vi "GUI_HTT_Switcher_tester.vi"() -> ()   [LabVIEW 2013]
uses:
  Shared/GUI_Template/GUI_master/tcp_new_data_event.ctl
  Shared/GUI_Template/GUI_master/tcp new data cluster.ctl
panel:
  in  "DigitalOutput.Channel 2::1":enum16{"on", "off"}(ring) caption="Phosphor"
  in  "Phosphor":bool
  in  "DigitalOutput.Channel 1::1":enum16{"on", "off"}(ring)
  in  "DigitalOutput.Channel 0::1":enum16{"on", "off"}(ring) caption="Flipper"
  in  "Flipper":bool
  out "error IO 2":errorcluster
  out "fire::10":string
  out "tcp data event":T1
  in  "UDP error message":string
  in  "GUIdevice 2":string
  in  "GUIdevice 1":string="HTT-Switch-DAQPad"
  in  "stop":bool
  # "Energy"
  # "HTT Switcher"
  # "In"
  # "Out"
  # "In"
  # "Out"
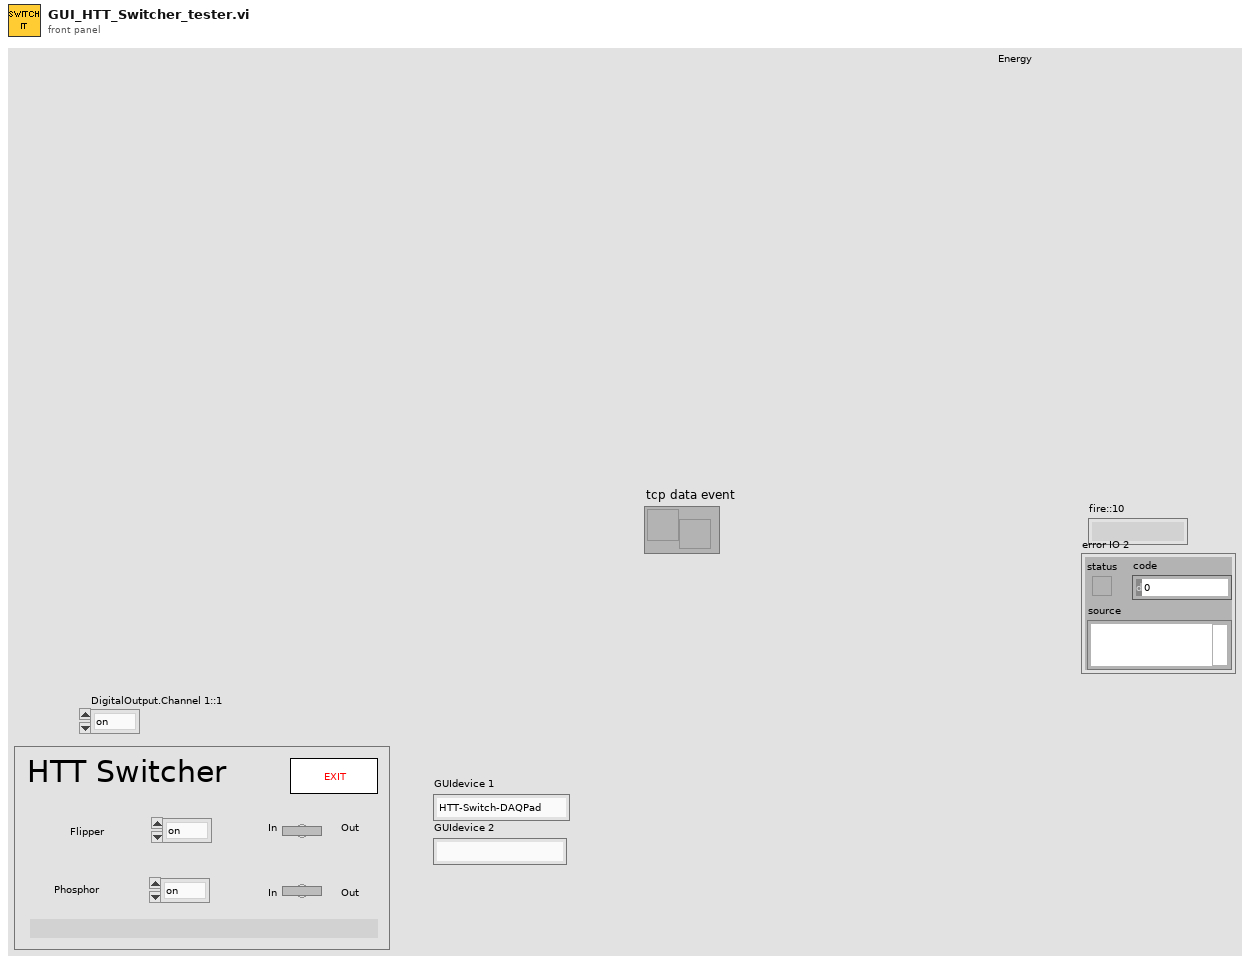
[diagram p1: front panel]
types:
  T1 = typedef "tcp_new_data_event.ctl" = refnum<user-event>
  T2 = typedef "tcp new data cluster.ctl" = cluster{"EventEnum":enum16{"new data", "connection status update"}, "Device name":string}
  T3 = enum32{"invalid app kind", "Development System", "Run Time System", "Student Edition", "Embedded LabVIEW", "Evaluation", "Custom"}
  T4 = enum32{"Invalid", "Standard", "Closed", "Hidden", "Minimized", "Maximized"}
  T5 = cluster{"Core":cluster{"Current VI Reference":refnum<vi>, "Close Panel on Exit?":bool}, "Heater timing offset":dbl, "Discharge timing offset":dbl, "irrelevant":bool, "Tik1":u32, "Tik2":u32, "notused":bool, "outoforder":bool, "notwhatyouthinkitis":enum16{"on", "off"}}
  T6 = cluster{"Current VI Reference":refnum<vi>, "Close Panel on Exit?":bool}
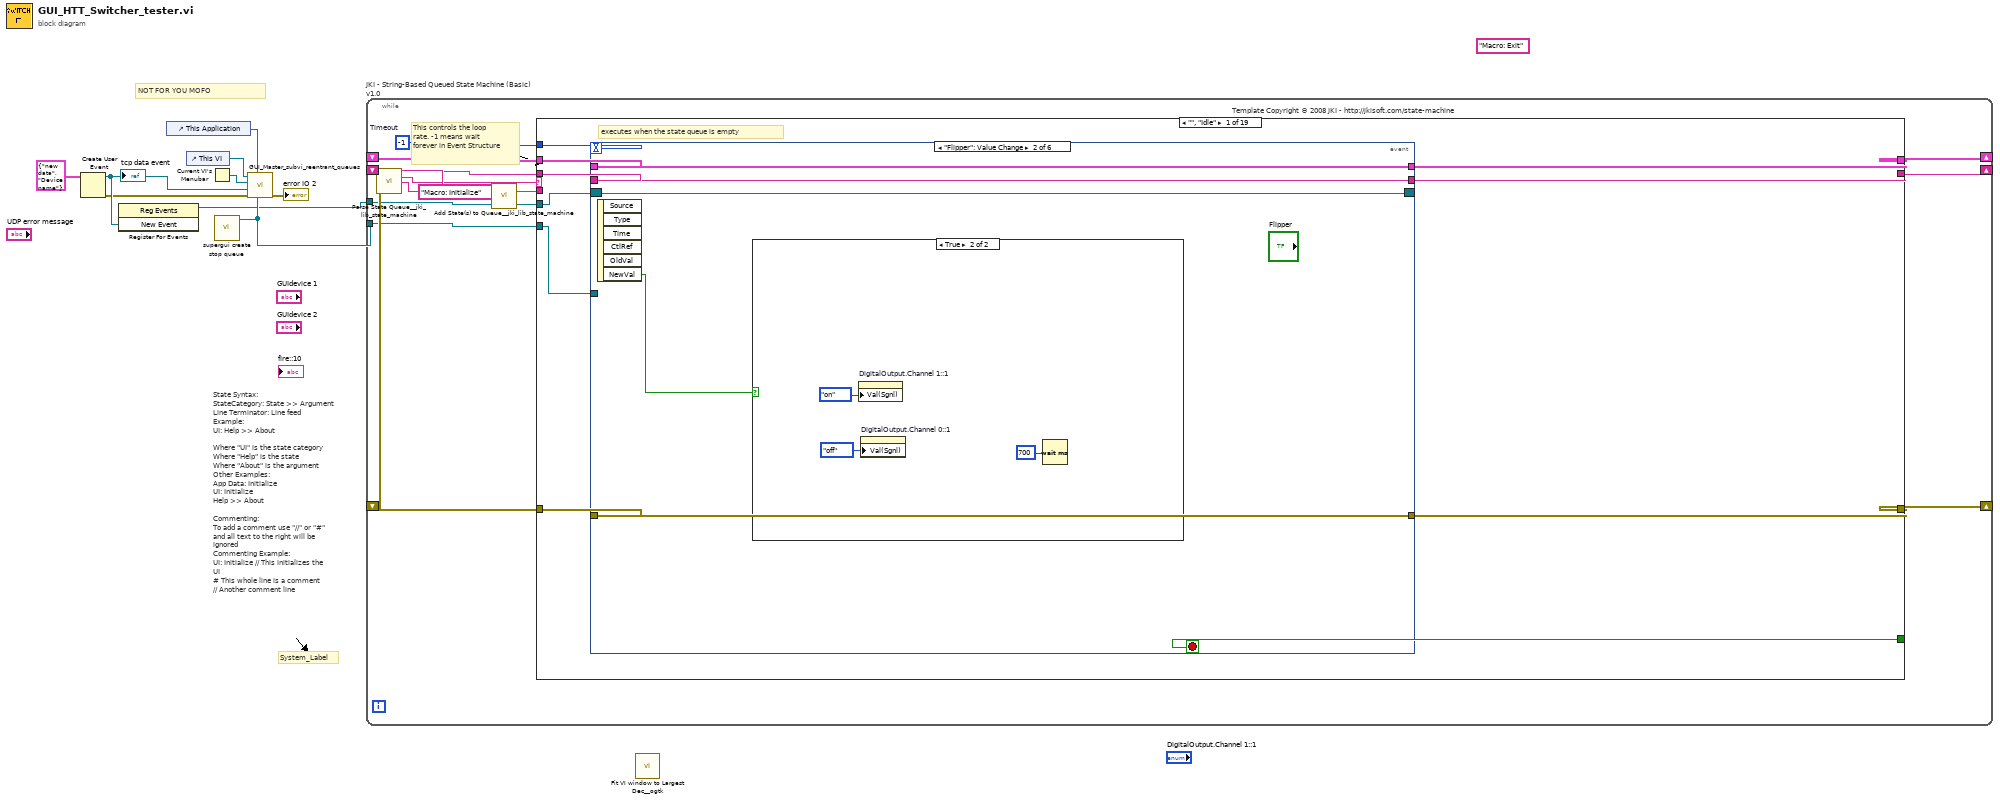
[diagram p0: block diagram]
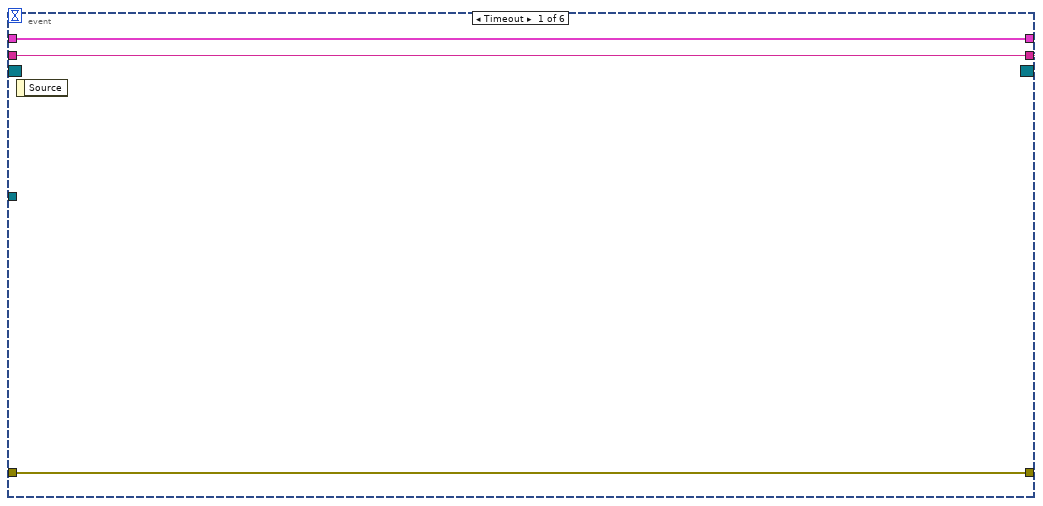
[diagram p2: hidden frame]
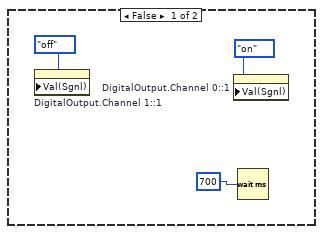
[diagram p3: hidden frame]
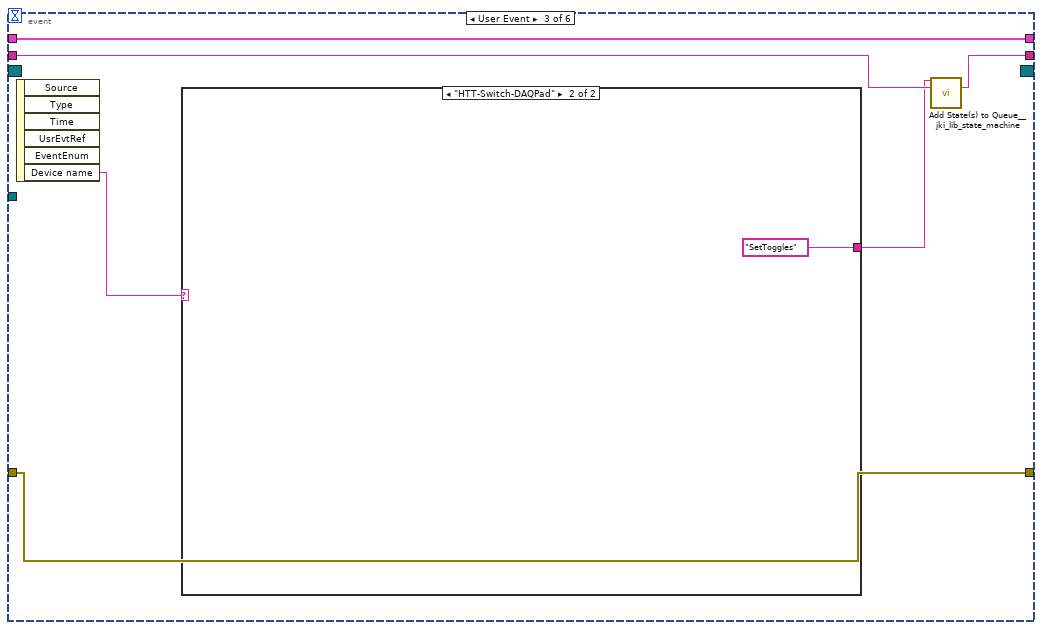
[diagram p4: hidden frame]
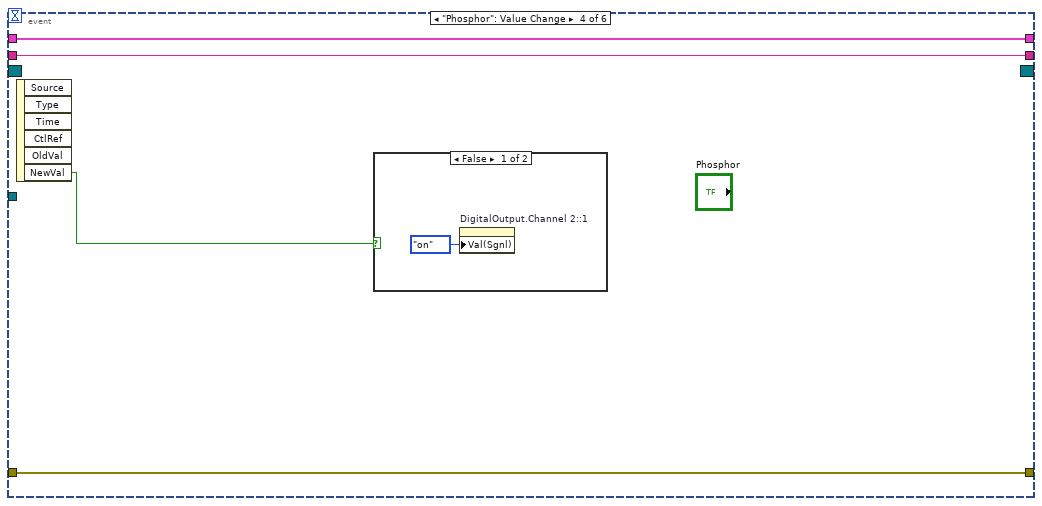
[diagram p6: hidden frame]
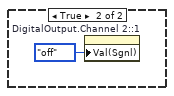
[diagram p7: hidden frame]
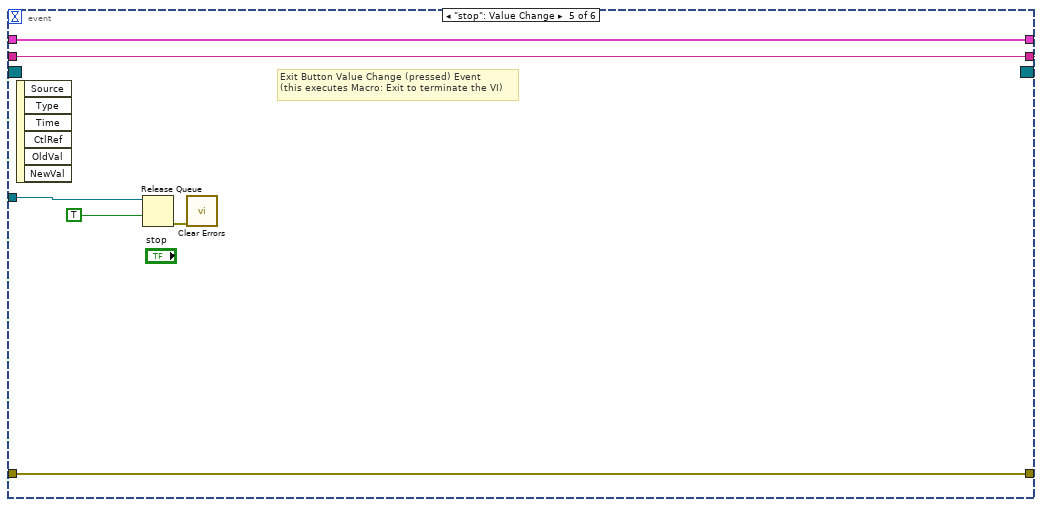
[diagram p8: hidden frame]
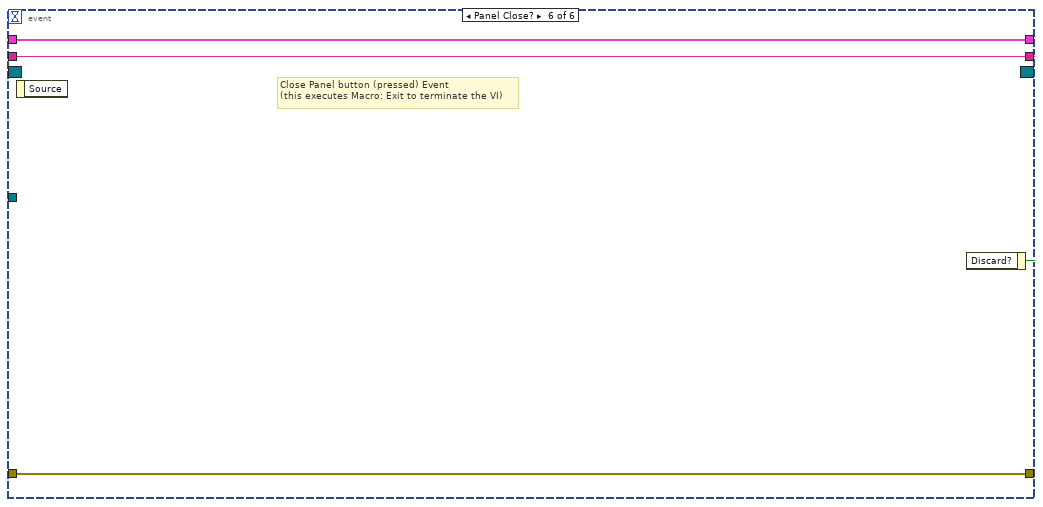
[diagram p9: hidden frame]
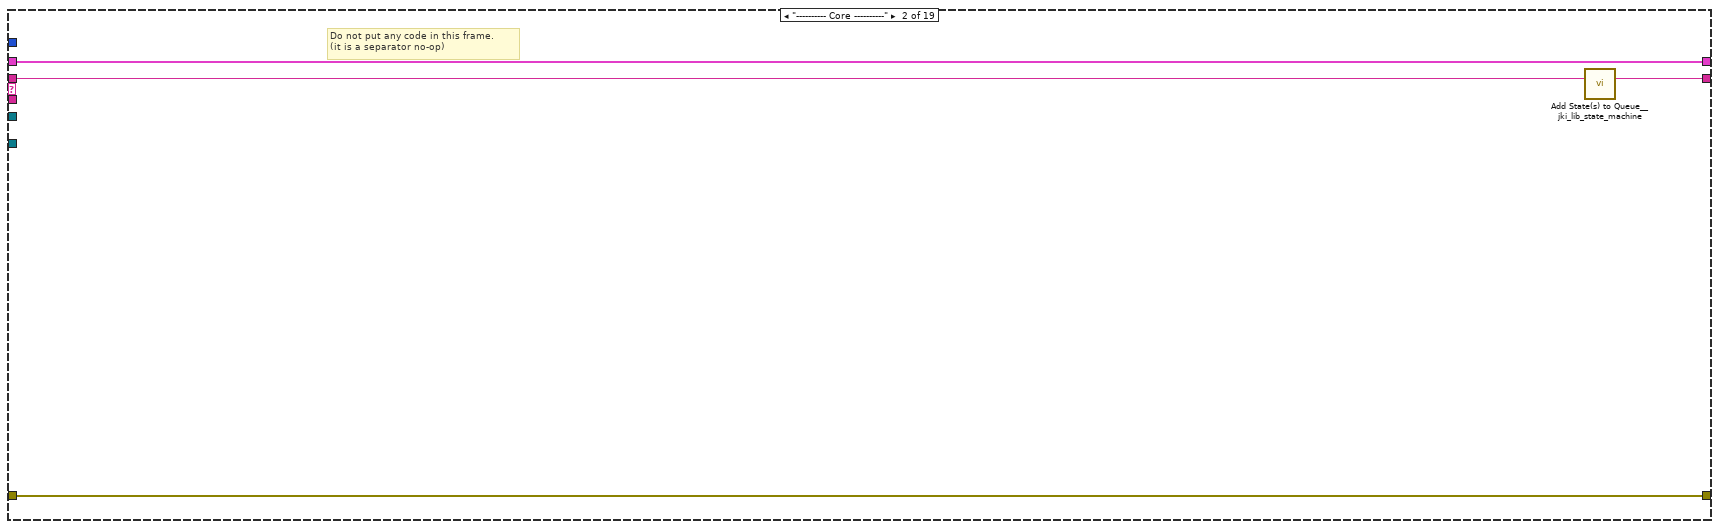
[diagram p10: hidden frame]
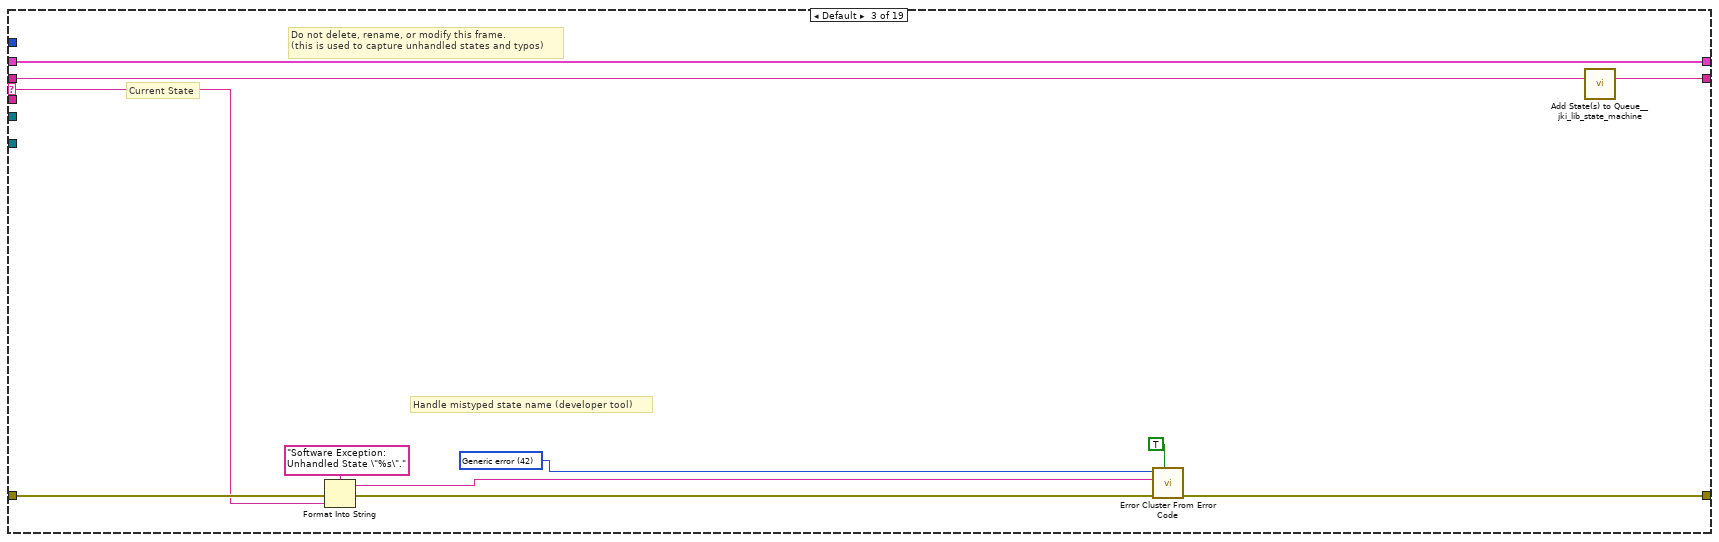
[diagram p11: hidden frame]
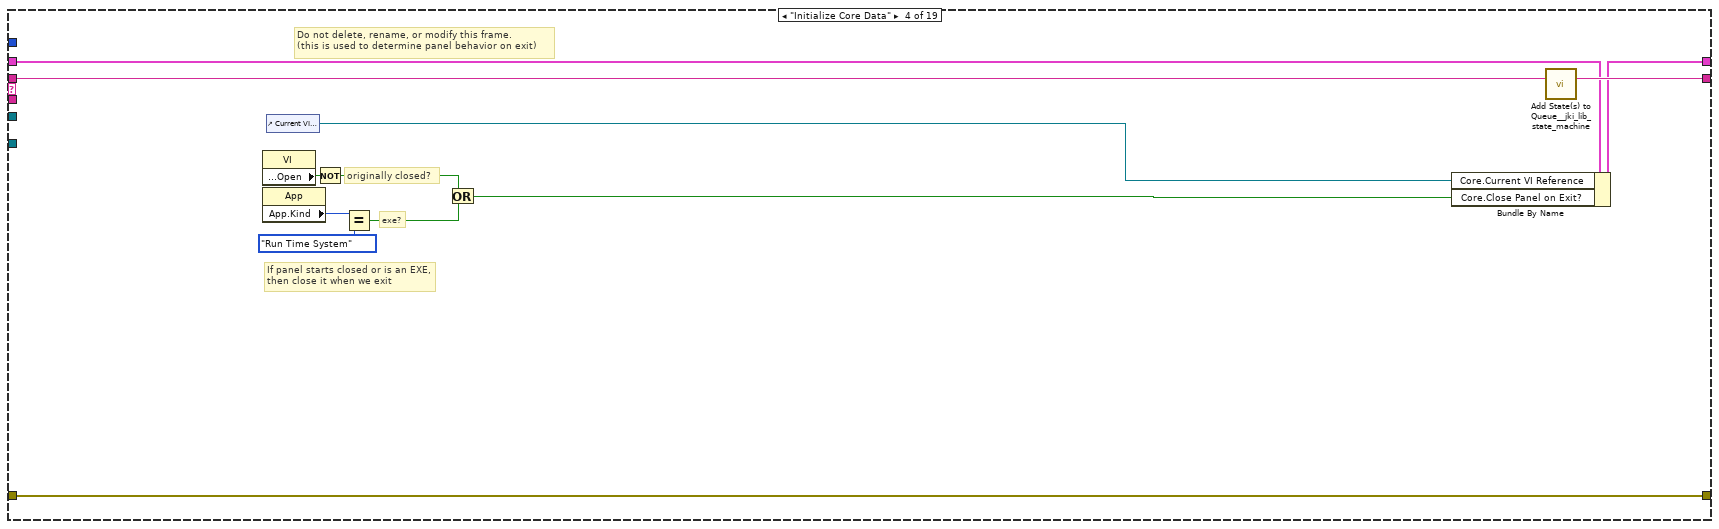
[diagram p12: hidden frame]
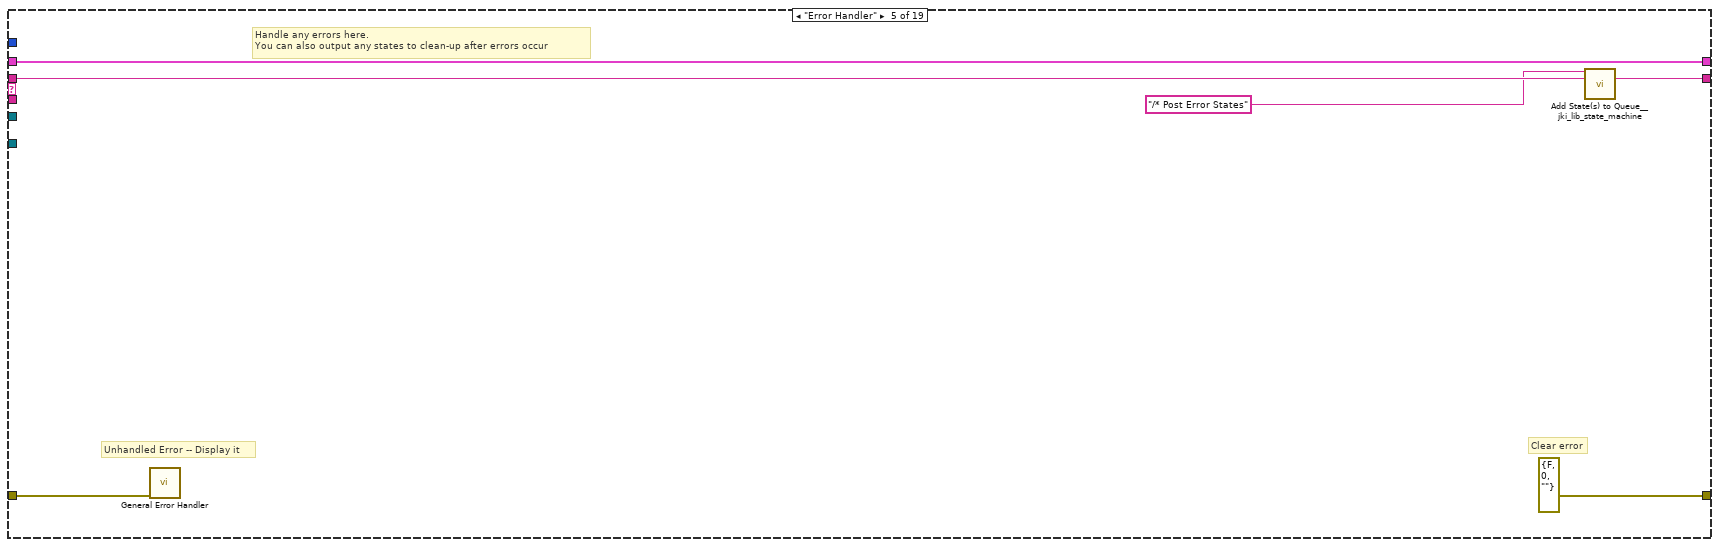
[diagram p13: hidden frame]
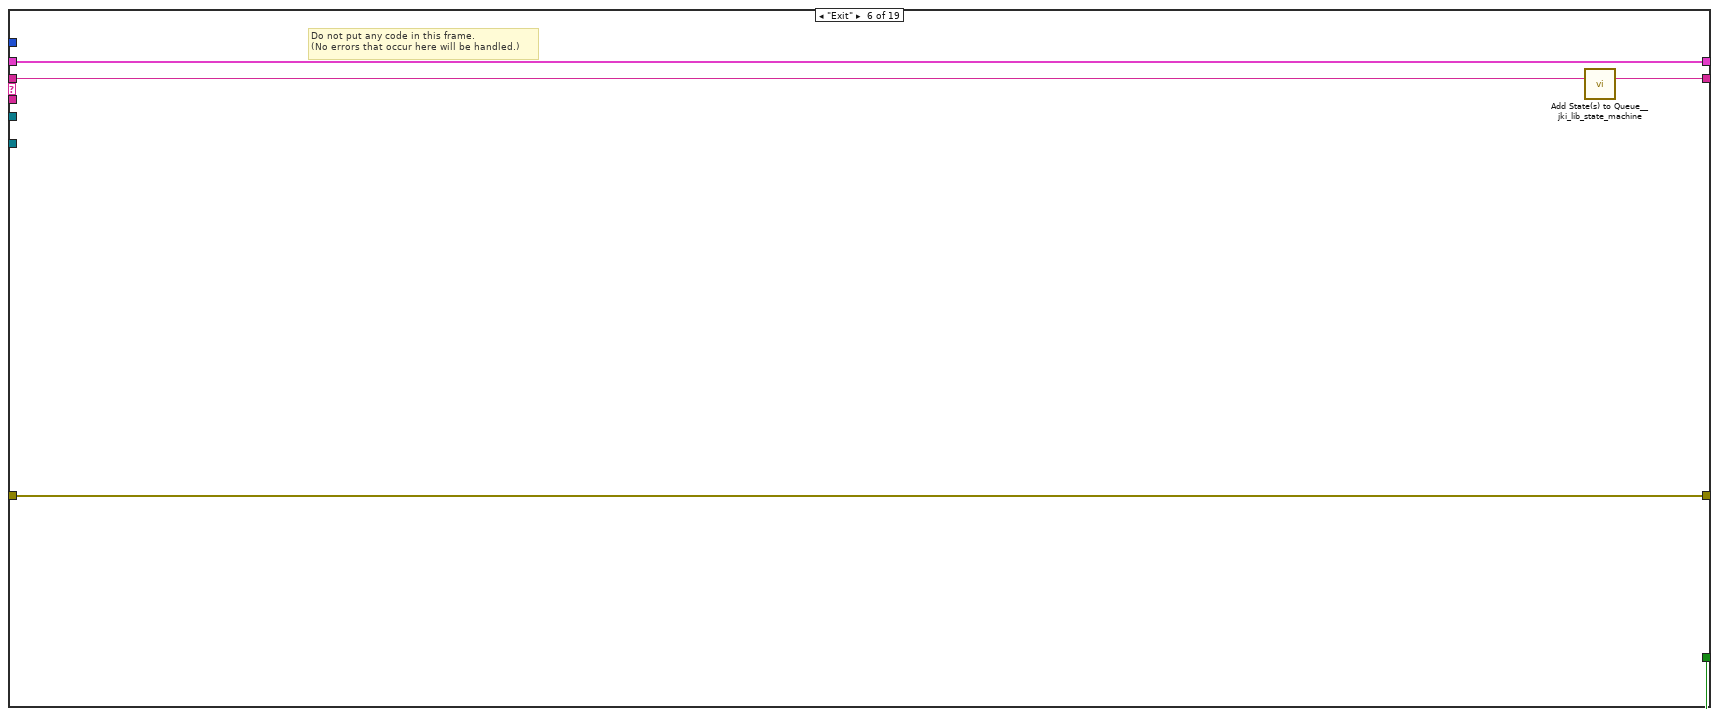
[diagram p14: hidden frame]
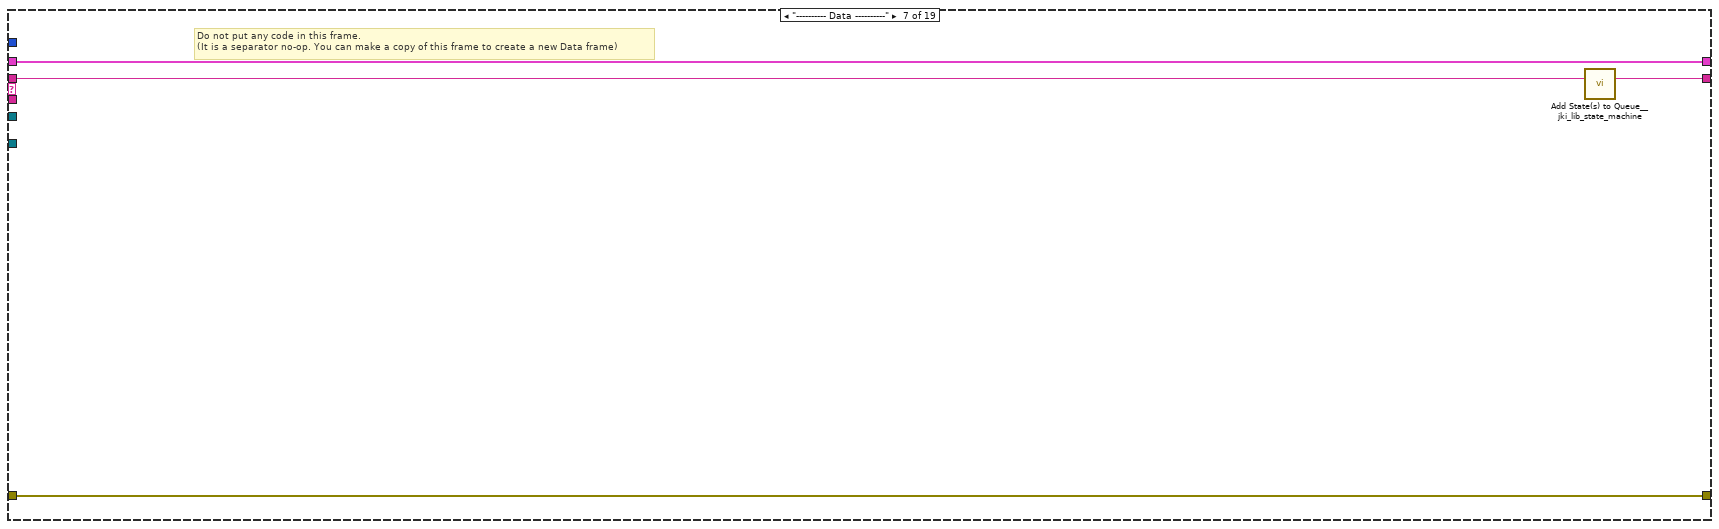
[diagram p15: hidden frame]
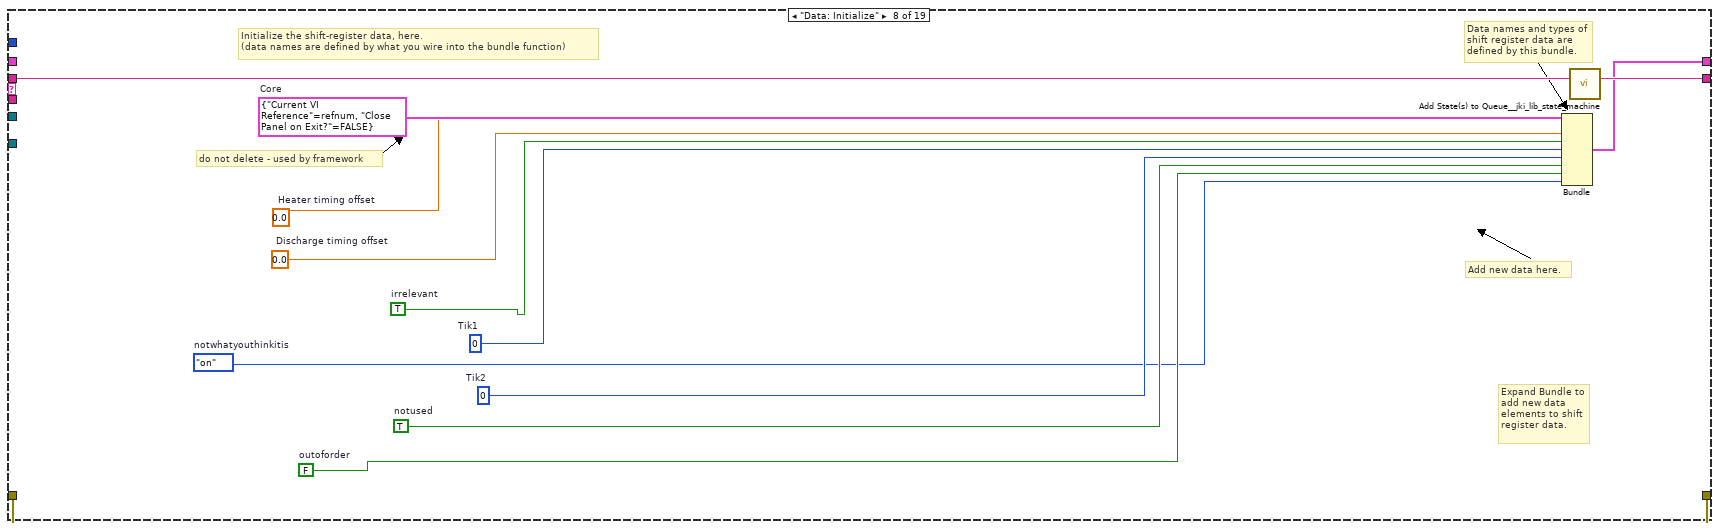
[diagram p16: hidden frame]
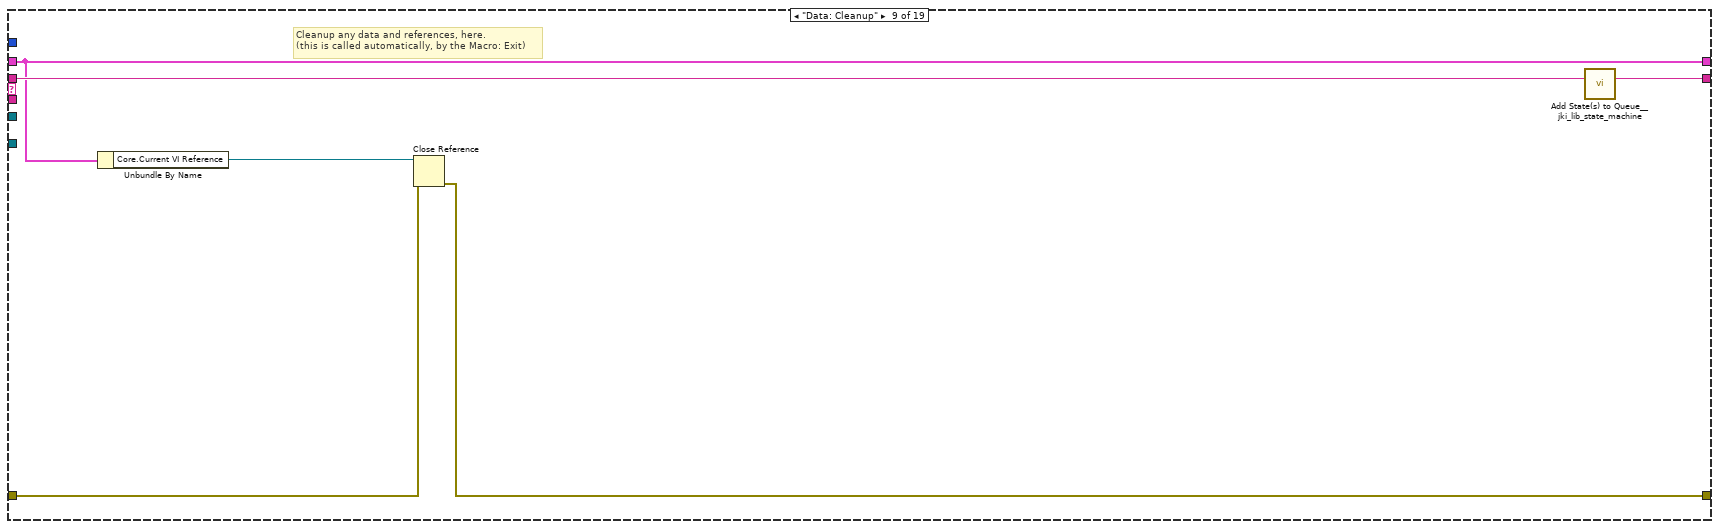
[diagram p17: hidden frame]
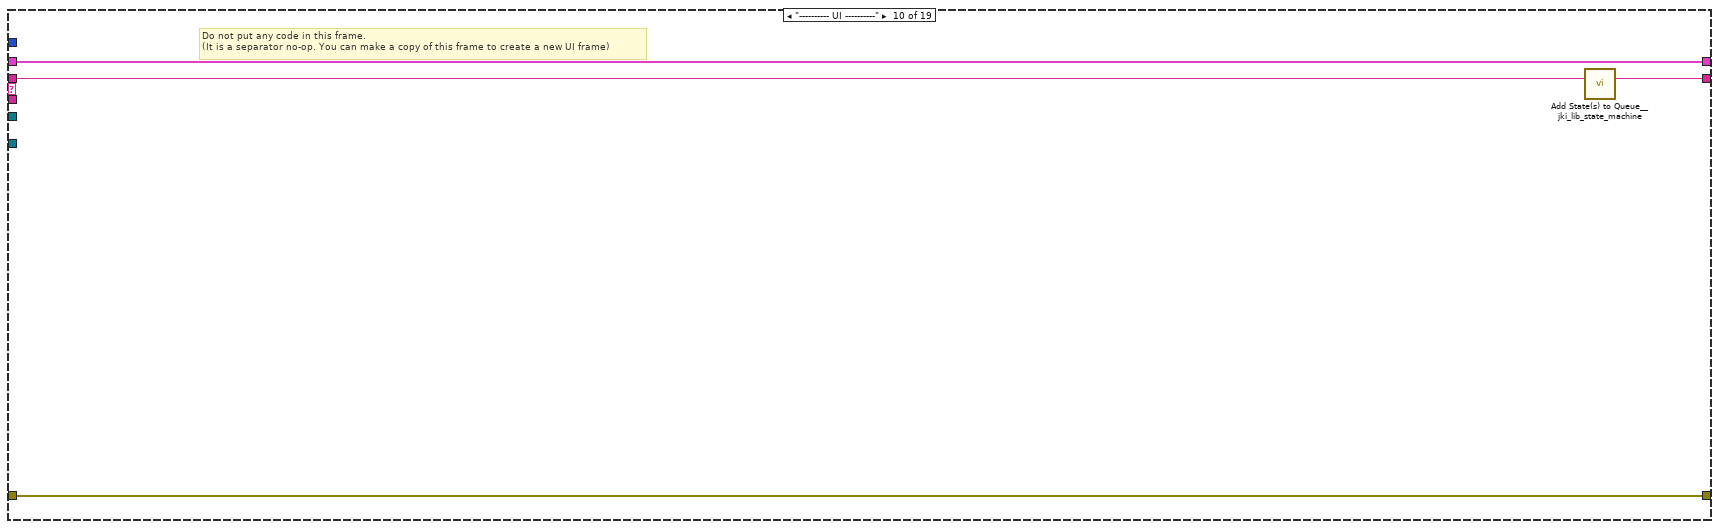
[diagram p18: hidden frame]
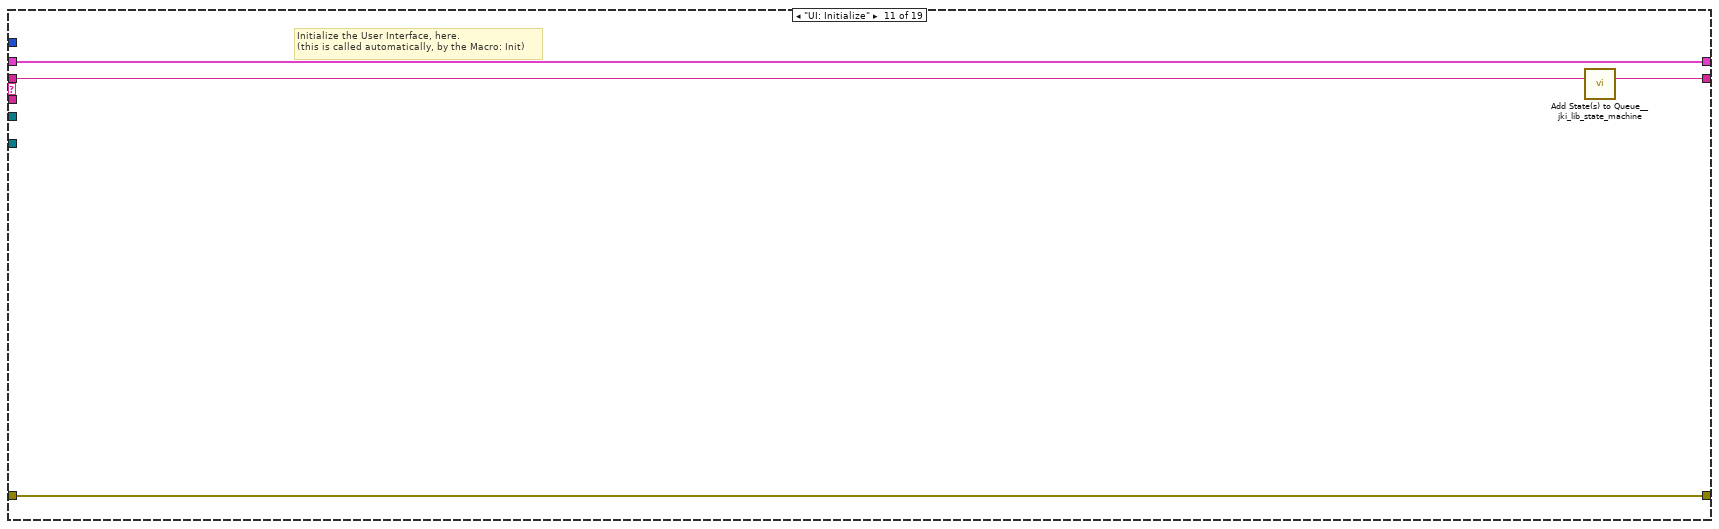
[diagram p19: hidden frame]
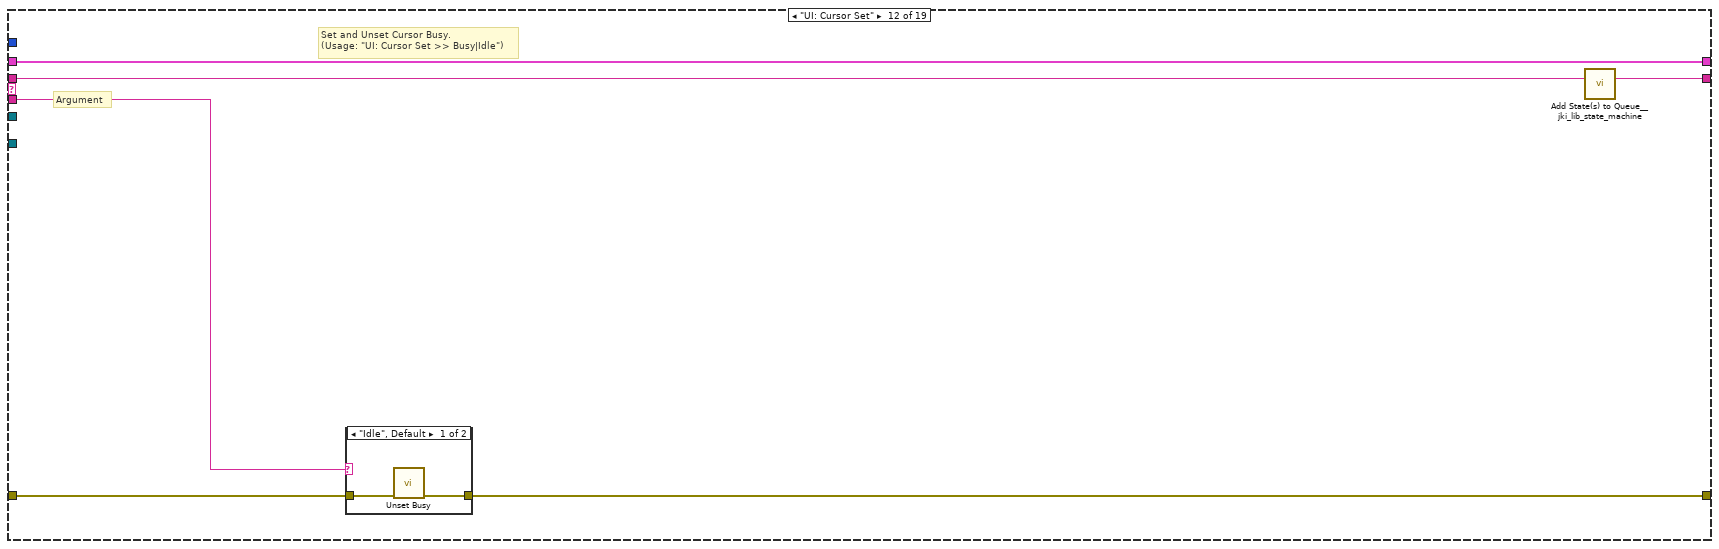
[diagram p20: hidden frame]
diagram:
  (unwired) "Macro: Exit"
  # "State Syntax:\nStateCategory: State >> Argument\nLine Terminator: Line feed\nExample:\nUI: Help >> About\n\nWhere \"UI\" is the state category\nWhere \"Help\" is the state\nWhere \"About\" is the argument\nOther Examples:\nApp Data: Initialize\nUI: Initialize\nHelp >> About\n\nCommenting:\nTo add a comment use \"//\" or \"#\" and all text to the right will be ignored\nCommenting Example:\nUI: Initialize // This initializes the UI\n# This whole line is a comment\n// Another comment line"
  # "This controls the loop rate. -1 means wait forever in Event Structure"
  # "System_Label"
  # "NOT FOR YOU MOFO"
  n1 = Create User Event(user event datatype=T2 {"EventEnum"=enum."new data", "Device name"="Device name"} ("New Event")) -> (user event=w10:refnum<user-event>, error out=w9:errorcluster)  [unwired: 1 in]
  "tcp data event" <- w10
  n2 = register-events(w10) -> (reference out=w1:refnum<event-registration>)  [unwired: 2 in, 1 out]
  n3 = control-ref of="This Application"() -> (w11:refnum<vi>)
  n4 = control-ref of="This VI"() -> (w5:refnum<vi>)
  n5 = Current VI's Menubar() -> (w7:refnum<k9>)
  n6 = call "supergui create stop queue.vi"() -> ("STOP Queue out"=w2:refnum<queue>)  [unwired: 11 in]
  n7 = call "GUI_Master_subvi_reentrant_queues.vi"("STOP Queue in"=w2, "This Application"=w11, "error in (no error)"=w9, "tcp data event"=w10, "Caller menu reference"=w7, "Caller VI ref"=w5) -> ("error out"=→"error IO 2":errorcluster)  [unwired: 5 in]
  n8 = call <vilib>:"Add State(s) to Queue__jki_lib_state_machine.vi"("State(s) in (\"\")"="Macro: Initialize") -> ("States Out"=w3:string)  [unwired: 14 in]
  n9 = while "JKI - String-Based Queued State Machine (Basic) v1.0" {
    shift-right: [w17] -> _
    shift-left: _ -> [w16]
    shift-right: [w20] -> _
    shift-left: _ -> [w14]
    shift-right: [w19] -> _
    shift-left: w3 -> [w21]
    tunnel: w1 -> [w13]
    tunnel: w2 -> [w12]
    stop <- w18 stop-if-true
    w15 = -1  # Timeout
    # "Template Copyright © 2008 JKI - http://jkisoft.com/state-machine"
    n10 = call <vilib>:"Parse State Queue__jki_lib_state_machine.vi"("State Queue"=w21, "Error In (no error)"=w14) -> ("Remaining States"=w23:string, "Current State"=w24:string, "Arguments"=w22:string)  [unwired: 11 in]
    n11 = case shown="\"\", \"Idle\"" w24 {
      selector: w24 -> [_ _ w80 _ _ _ _ _ _ _ _ _ _ _ _ _ _ _ _]
      tunnel: w23 -> [w33 w79 w84 w102 w108 w113 w117 w130 w136 w140 w144 w150 w161 w187 w192 w202 w206 w212 w220]
      tunnel: w22 -> [_ _ _ _ _ _ _ _ _ _ _ w145 w155 _ _ _ _ _ _]
      tunnel: w16 -> [w31 w76 w82 w93 w105 w111 w114 _ w131 w137 w142 w148 w157 w184 w188 w199 w203 w210 w215]
      tunnel: [w30 w77 w86 w99 errorcluster {"status"=FALSE, "code"=0, "source"=""} ("error out") w110 w115 w127 w132 w138 w141 w146 w158 w185 w190 w200 w204 w207 w216] -> w20
      tunnel: w14 -> [w29 w77 w85 w99 w104 w110 w115 w127 w133 w138 w141 w147 w159 w185 w190 w200 w204 w208 w216]
      tunnel: [w32 w78 w83 w101 w107 w112 w116 w129 w135 w139 w143 w149 w160 w186 w191 w201 w205 w211 w219] -> w19
      tunnel: [_ _ _ _ _ TRUE _ _ _ _ _ _ _ _ _ _ _ _ _] -> w18
      tunnel: [w25 w76 w82 w100 w105 w111 w114 w128 w131 w137 w142 w148 w157 w184 w188 w199 w203 w210 w215] -> w17
      tunnel: w15 -> [w28 _ _ _ _ _ _ _ _ _ _ _ _ _ _ _ _ _ _]
      tunnel: w13 -> [w27 _ _ _ _ _ _ _ _ _ _ _ _ _ _ _ _ _ _]
      tunnel: w12 -> [w26 _ _ _ _ _ _ _ _ _ _ _ _ _ _ _ _ _ _]
      frame "", "Idle" {
        # "executes when the state queue is empty"
        n12 = event shown="[1] \"Flipper\": Value Change" {
          selector: w27 -> [_ w41 _ _ _ _]
          dyn-events: [_ w41 _ _ _ _] -> _
          timeout: w28 -> [_ _ _ _ _ _]
          tunnel: w33 -> [w37 w42 w51 w59 w69 w75]
          tunnel: [w36 w42 w50 w59 w68 w74] -> w32
          tunnel: w31 -> [w34 w38 w53 w56 w66 w72]
          tunnel: [w35 w40 w52 w58 w67 w73] -> w30
          tunnel: w29 -> [w35 w40 w52 w58 w67 w73]
          tunnel: w26 -> [_ _ _ _ w63 _]
          tunnel: [w34 w38 w53 w56 w66 w72] -> w25
          event Timeout {
            n13 = event-data() -> ()  [unwired: 1 in, 1 out]
            n14 = call <vilib>:"Add State(s) to Queue__jki_lib_state_machine.vi"("State(s) in (\"\")"=w37) -> ("States Out"=w36:string)  [unwired: 14 in]
          }
          event "Flipper": Value Change {
            n15 = event-data() -> ("NewVal"=w39:bool)  [unwired: 1 in, 5 out]
            n16 = case shown="True" w39 {
              frame False {
                n17 = property on="DigitalOutput.Channel 1::1" class="Enum (strict)"("Val(Sgnl)"=enum16{"on", "off"}."off" ("Value (Signaling)")) -> ()  [unwired: 2 in, 2 out]
                n18 = property on="DigitalOutput.Channel 0::1" class="Enum (strict)"("Val(Sgnl)"=enum16{"on", "off"}."on" ("Value (Signaling)")) -> ()  [unwired: 2 in, 2 out]
                n19 = Wait (ms)(milliseconds to wait=u32 700) -> ()  [unwired: 1 out]
              }
              frame True {
                n20 = property on="DigitalOutput.Channel 1::1" class="Enum (strict)"("Val(Sgnl)"=enum16{"on", "off"}."on" ("Value (Signaling)")) -> ()  [unwired: 2 in, 2 out]
                n21 = property on="DigitalOutput.Channel 0::1" class="Enum (strict)"("Val(Sgnl)"=enum16{"on", "off"}."off" ("Value (Signaling)")) -> ()  [unwired: 2 in, 2 out]
                n22 = Wait (ms)(milliseconds to wait=u32 700) -> ()  [unwired: 1 out]
              }
            }
          }
          event User Event {
            n23 = event-data() -> ("Device name"=w54:string)  [unwired: 1 in, 5 out]
            n24 = case shown="\"HTT-Switch-DAQPad\"" w54 {
              tunnel: [_ "SetToggles"] -> w49
              frame "False", Default {
              }
              frame "HTT-Switch-DAQPad" {
              }
            }
            n25 = call <vilib>:"Add State(s) to Queue__jki_lib_state_machine.vi"("State(s) in Front (\"\")"=w49, "State(s) in (\"\")"=w51) -> ("States Out"=w50:string)  [unwired: 13 in]
          }
          event "Phosphor": Value Change {
            n26 = event-data() -> ("NewVal"=w57:bool)  [unwired: 1 in, 5 out]
            n27 = case shown="False" w57 {
              frame False {
                n28 = property on="DigitalOutput.Channel 2::1" class="Enum (strict)"("Val(Sgnl)"=enum16{"on", "off"}."on" ("Value (Signaling)")) -> ()  [unwired: 2 in, 2 out]
              }
              frame True {
                n29 = property on="DigitalOutput.Channel 2::1" class="Enum (strict)"("Val(Sgnl)"=enum16{"on", "off"}."off" ("Value (Signaling)")) -> ()  [unwired: 2 in, 2 out]
              }
            }
          }
          event "stop": Value Change {
            # "Exit Button Value Change (pressed) Event\n(this executes Macro: Exit to terminate the VI)"
            n30 = event-data() -> ()  [unwired: 1 in, 6 out]
            n31 = Release Queue(queue=w63, force destroy? (F)=TRUE) -> (error out=w64:errorcluster)  [unwired: 1 in, 2 out]
            n32 = call <vilib>:"Clear Errors.vi"("error in (no error)"=w64) -> ()  [unwired: 6 in, 1 out]
            n33 = call <vilib>:"Add State(s) to Queue__jki_lib_state_machine.vi"("State(s) in Front (\"\")"="Macro: Exit", "State(s) in (\"\")"=w69) -> ("States Out"=w68:string)  [unwired: 13 in]
          }
          event Panel Close? {
            # "Discard the event because we'll close the front panel ourselves in Macro: Exit"
            # "Close Panel button (pressed) Event\n(this executes Macro: Exit to terminate the VI)"
            n34 = event-data() -> ()  [unwired: 1 in, 1 out]
            n35 = event-data("Discard?"=TRUE) -> ()  [unwired: 1 in, 1 out]
            n36 = call <vilib>:"Add State(s) to Queue__jki_lib_state_machine.vi"("State(s) in Front (\"\")"="Macro: Exit", "State(s) in (\"\")"=w75) -> ("States Out"=w74:string)  [unwired: 13 in]
          }
        }
      }
      frame "---------- Core ----------" {
        # "Do not put any code in this frame.\n(it is a separator no-op)"
        n37 = call <vilib>:"Add State(s) to Queue__jki_lib_state_machine.vi"("State(s) in (\"\")"=w79) -> ("States Out"=w78:string)  [unwired: 14 in]
      }
      frame Default {
        w89 = 42 items=["No error", "Argument error", "Memory is full", "Out of zone", "End of file", "File already open", "Generic file I/O error", "File not found", "File permission error", "Disk is full", "Duplicate path", "Too many files open", "System feature not enabled", "Resource file not found", "Cannot add resource", "Resource not found", "Image not found", "Image memory error", "Pen does not exist", "Config type invalid", "Config token not found", "Config parse error", "Config memory error", "Bad external code format", "Bad external code offset", "External code not present", "Null window", "Destroy window error", "Null menu", "Print aborted", "Bad print record", "Print driver error", "Windows error during printing", "Memory error during printing", "Print dialog error", "Generic print error", "Invalid device refnum", "Device not found", "Device parameter error", "Device unit error", "Cannot open device", "Device call aborted", "Generic error", "Cancelled by user", "Object ID too low", "Object ID too high", "Object not in heap", "Unknown heap", "Unknown object (invalid DefProc)", "Unknown object (DefProc not in table)", "Message out of range", "Invalid (null) method", "Unknown message", "Manager call not supported", "Bad address", "Network operation in progress", "Network operation timed out", "Connection is busy", "Network attribute not supported", "Network error", "Address in use", "System out of memory", "Connection aborted", "Connection refused", "Not connected", "Already connected", "Connection closed", "Initialization error (interapplication manager)", "Bad occurrence", "Wait on unbound occurrence handler", "Occurrence queue overflow", "Datalog type conflict", "Unused", "Unrecognized type (interapplication manager)", "Memory corrupt", "Failed to make temporary DLL", "Old CIN version", "Drag socket not found", "Failed to load drop-object", "Failed to register OLE object", "Failed to release OLE object", "Format specifier type mismatch", "Unknown format specifier", "Too few format specifiers", "Too many format specifiers", "Scan failed", "Newer CIN version", "Error converting to variant", "Runtime menu error", "Password tampered", "Variant attribute not found", "Incompatible variant data type", "Event data is not available", "Event Store is not present", "Occurrence is not found", "Event Queue is not created", "Event info is not available", "Refnum passed is NULL", "Error retrieving Class GUID", "Error retrieving CoClass GUID", "Error retrieving TypeLib GUID.", "Bad built application magic bytes.", "Specific driver is different from the specific driver associated with the Logical Name.", "There is no session opened to the class driver.", "Max Error", "MAX - Error with config objects", "MAX - Error loading configuration", "MAX - Group not supported"]
        # "Current State"
        # "Do not delete, rename, or modify this frame.\n(this is used to capture unhandled states and typos)"
        # "Handle mistyped state name (developer tool)"
        n38 = Format Into String(format string="Software Exception: Unhandled State \"%s\"." ("message"), error in=w85, w80) -> (resulting string=w88:string, error out=w87:errorcluster)  [unwired: 1 in]
        n39 = call <vilib>:"Error Cluster From Error Code.vi"("show call chain? (False)"=TRUE, "error in (no error)"=w87, "error message (\"\")"=w88, "error code (0)"=w89) -> ("error out"=w86:errorcluster)  [unwired: 5 in]
        n40 = call <vilib>:"Add State(s) to Queue__jki_lib_state_machine.vi"("State(s) in (\"\")"=w84) -> ("States Out"=w83:string)  [unwired: 14 in]
      }
      frame "Initialize Core Data" {
        # "Do not delete, rename, or modify this frame.\n(this is used to determine panel behavior on exit)"
        # "originally closed?"
        # "exe?"
        # "If panel starts closed or is an EXE, then close it when we exit"
        n41 = property class="VI"() -> ("Front Panel.Open"=w98:bool)  [unwired: 2 in, 2 out]
        n42 = property class="App"() -> ("App.Kind"=w97:T3)  [unwired: 2 in, 2 out]
        n43 = control-ref of="Current VI Reference"() -> (w91:refnum<vi>)
        n44 = Not(x=w98) -> (.not. x?=w95:bool)
        n45 = Equal?(x=w97, y=T3."Run Time System" ("Application:Kind")) -> (x = y?=w94:bool)
        n46 = Or(x=w95, y=w94) -> (x .or. y?=w92:bool)
        n47 = Bundle By Name(cluster=w93, "Core.Current VI Reference"=w91, "Core.Close Panel on Exit?"=w92) -> (w100:T5)
        n48 = call <vilib>:"Add State(s) to Queue__jki_lib_state_machine.vi"("State(s) in (\"\")"=w102) -> ("States Out"=w101:string)  [unwired: 14 in]
      }
      frame "Error Handler" {
        # "Unhandled Error -- Display it"
        # "Handle any errors here.\nYou can also output any states to clean-up after errors occur"
        # "Clear error"
        n49 = call <vilib>:"General Error Handler.vi"("error in (no error)"=w104) -> ()  [unwired: 10 in, 5 out]
        n50 = call <vilib>:"Add State(s) to Queue__jki_lib_state_machine.vi"("State(s) in Front (\"\")"="/* Post Error States", "State(s) in (\"\")"=w108) -> ("States Out"=w107:string)  [unwired: 13 in]
      }
      frame "Exit" {
        # "Do not put any code in this frame.\n(No errors that occur here will be handled.)"
        n51 = call <vilib>:"Add State(s) to Queue__jki_lib_state_machine.vi"("State(s) in (\"\")"=w113) -> ("States Out"=w112:string)  [unwired: 14 in]
      }
      frame "---------- Data ----------" {
        # "Do not put any code in this frame.\n(It is a separator no-op. You can make a copy of this frame to create a new Data frame)"
        n52 = call <vilib>:"Add State(s) to Queue__jki_lib_state_machine.vi"("State(s) in (\"\")"=w117) -> ("States Out"=w116:string)  [unwired: 14 in]
      }
      frame "Data: Initialize" {
        w118 = enum16{"on", "off"}."on"  # notwhatyouthinkitis
        w119 = FALSE  # outoforder
        w120 = TRUE  # irrelevant
        w121 = TRUE  # notused
        w123 = u32 0  # Tik1
        w122 = u32 0  # Tik2
        w124 = 0.0  # Discharge timing offset
        w125 = 0.0  # Heater timing offset
        w126 = T6 {"Current VI Reference"=refnum, "Close Panel on Exit?"=FALSE}  # Core
        # "do not delete - used by framework"
        # "Expand Bundle to add new data elements to shift register data."
        # "Add new data here."
        # "Data names and types of shift register data are defined by this bundle."
        # "Initialize the shift-register data, here.\n(data names are defined by what you wire into the bundle function)"
        n53 = Bundle("Core"=w126, "Heater timing offset"=w125, "Discharge timing offset"=w124, "irrelevant"=w120, "Tik1"=w123, "Tik2"=w122, "notused"=w121, "outoforder"=w119, "notwhatyouthinkitis"=w118) -> (w128:T5)  [unwired: 1 in]
        n54 = call <vilib>:"Add State(s) to Queue__jki_lib_state_machine.vi"("State(s) in (\"\")"=w130) -> ("States Out"=w129:string)  [unwired: 14 in]
      }
      frame "Data: Cleanup" {
        # "Cleanup any data and references, here.\n(this is called automatically, by the Macro: Exit)"
        n55 = Unbundle By Name(w131) -> ("Core.Current VI Reference"=w134:refnum<vi>)
        n56 = Close Reference(reference=w134, error in (no error)=w133) -> (error out=w132:errorcluster)
        n57 = call <vilib>:"Add State(s) to Queue__jki_lib_state_machine.vi"("State(s) in (\"\")"=w136) -> ("States Out"=w135:string)  [unwired: 14 in]
      }
      frame "---------- UI ----------" {
        # "Do not put any code in this frame.\n(It is a separator no-op. You can make a copy of this frame to create a new UI frame)"
        n58 = call <vilib>:"Add State(s) to Queue__jki_lib_state_machine.vi"("State(s) in (\"\")"=w140) -> ("States Out"=w139:string)  [unwired: 14 in]
      }
      frame "UI: Initialize" {
        # "Initialize the User Interface, here.\n(this is called automatically, by the Macro: Init)"
        n59 = call <vilib>:"Add State(s) to Queue__jki_lib_state_machine.vi"("State(s) in (\"\")"=w144) -> ("States Out"=w143:string)  [unwired: 14 in]
      }
      frame "UI: Cursor Set" {
        # "Argument"
        # "Set and Unset Cursor Busy.\n(Usage: \"UI: Cursor Set >> Busy|Idle\")"
        n60 = case shown="\"Idle\", Default" w145 {
          tunnel: w147 -> [w152 w154]
          tunnel: [w151 w153] -> w146
          frame "Idle", Default {
            n61 = call <vilib>:"Unset Busy.vi"("error in (no error)"=w152) -> ("error out"=w151:errorcluster)  [unwired: 10 in]
          }
          frame "Busy" {
            n62 = call <vilib>:"Set Busy.vi"("error in (no error)"=w154) -> ("error out"=w153:errorcluster)  [unwired: 9 in, 1 out]
          }
        }
        n63 = call <vilib>:"Add State(s) to Queue__jki_lib_state_machine.vi"("State(s) in (\"\")"=w150) -> ("States Out"=w149:string)  [unwired: 14 in]
      }
      frame "UI: Front Panel State" {
        # "Argument"
        # "Set Front Panel Open or Closed\n(Usage: \"UI: Front Panel State >> Open|Close\")"
        n64 = Unbundle By Name(w157) -> ("Core.Current VI Reference"=w156:refnum<vi>)
        n65 = case shown="\"Close\"" w155 {
          tunnel: w159 -> [w165 w178]
          tunnel: [w167 w179] -> w158
          tunnel: w156 -> [w166 w176]
          frame "Open", Default {
            n66 = property class="VI"(reference=w166, error in=w165) -> (reference out=w163:refnum<vi>, error out=w164:errorcluster, "Front Panel.Open"=w162:bool)
            n67 = case shown="False" w162 {
              tunnel: [w170 w173] -> w167
              tunnel: w164 -> [w169 w173]
              tunnel: w163 -> [w168 _]
              frame False {
                n68 = invoke class="VI" method="FP.Open"(reference=w168, error in=w169, "Activate"=TRUE, "State"=T4."Standard") -> (error out=w170:errorcluster)  [unwired: 1 in, 4 out]
              }
              frame True {
              }
            }
          }
          frame "Close" {
            n69 = property class="VI"(reference=w176, error in=w178) -> (reference out=w175:refnum<vi>, error out=w177:errorcluster, "Front Panel.Open"=w174:bool)
            n70 = case shown="True" w174 {
              tunnel: [w180 w183] -> w179
              tunnel: w177 -> [w180 w182]
              tunnel: w175 -> [_ w181]
              frame False {
              }
              frame True {
                n71 = invoke class="VI" method="FP.Close"(reference=w181, error in=w182) -> (error out=w183:errorcluster)  [unwired: 1 in, 2 out]
              }
            }
          }
        }
        n72 = call <vilib>:"Add State(s) to Queue__jki_lib_state_machine.vi"("State(s) in (\"\")"=w161) -> ("States Out"=w160:string)  [unwired: 14 in]
      }
      frame "---------- Macro ----------" {
        # "Do not put any code in this frame.\n(It is a separator no-op. You can make a copy of this frame to create a new Macro frame)"
        n73 = call <vilib>:"Add State(s) to Queue__jki_lib_state_machine.vi"("State(s) in (\"\")"=w187) -> ("States Out"=w186:string)  [unwired: 14 in]
      }
      frame "Macro: Initialize" {
        w189 = "Data: Initialize\nInitialize Core Data\nUI: Initialize\nUI: Front Panel State >> Open"  # Data: Initialize Initialize Core Data UI: Initialize UI: Front Panel State >> Open
        # "Initialization Macro\n(This is called once, when the VI starts)"
        n74 = call <vilib>:"Add State(s) to Queue__jki_lib_state_machine.vi"("State(s) in Front (\"\")"=w189, "State(s) in (\"\")"=w192) -> ("States Out"=w191:string)  [unwired: 13 in]
      }
      frame "Macro: Exit" {
        # "Exit Macro\n(This is called once, when the VI exits)"
        n75 = Unbundle By Name(w199) -> ("Core.Close Panel on Exit?"=w198:bool)
        n76 = Select(t="UI: Front Panel State >> Close", s=w198, f="") -> (s? t:f=w195:string)
        n77 = call <vilib>:"Add State(s) to Queue__jki_lib_state_machine.vi"("State(s) in (\"\")"=w195, "State(s) at Back (\"\")"="Data: Cleanup\nExit") -> ("States Out"=w193:string)  [unwired: 13 in]
        n78 = call <vilib>:"Add State(s) to Queue__jki_lib_state_machine.vi"("State(s) in Front (\"\")"=w193, "State(s) in (\"\")"=w202) -> ("States Out"=w201:string)  [unwired: 13 in]
      }
      frame "---------- New Category ----------" {
        # "Template Separator\n(You can make a copy of, or modify, this frame)"
        n79 = call <vilib>:"Add State(s) to Queue__jki_lib_state_machine.vi"("State(s) in (\"\")"=w206) -> ("States Out"=w205:string)  [unwired: 14 in]
      }
      frame "Action: Fire" {
        # "Your code here.\n(You can make a copy of, or modify, this frame)"
        n80 = property on="fire::10" class="Str"(error in=w208, "Val(Sgnl)"="fire>>force" ("Value (Signaling)")) -> (error out=w207:errorcluster)  [unwired: 1 in, 1 out]
        n81 = call <vilib>:"Add State(s) to Queue__jki_lib_state_machine.vi"("State(s) in (\"\")"=w212) -> ("States Out"=w211:string)  [unwired: 14 in]
      }
      frame "SetToggles" {
        # "Your code here.\n(You can make a copy of, or modify, this frame)"
        n82 = case shown="\"off\"" "DigitalOutput.Channel 2::1" {
          tunnel: [FALSE ("Phosphor") TRUE ("Phosphor")] -> w217
          frame "on", Default {
          }
          frame "off" {
          }
        }
        n83 = case shown="\"off\"" "DigitalOutput.Channel 0::1" {
          tunnel: [FALSE ("Flipper") TRUE ("Flipper")] -> w213
          frame "on", Default {
          }
          frame "off" {
          }
        }
        n84 = local write "Phosphor"(w217) -> ()
        n85 = local write "Flipper"(w213) -> ()
        n86 = call <vilib>:"Add State(s) to Queue__jki_lib_state_machine.vi"("State(s) in (\"\")"=w220) -> ("States Out"=w219:string)  [unwired: 14 in]
      }
    }
  }
  n87 = call <userlib>:"Fit VI window to Largest Dec__ogtk.vi"() -> ()  [unwired: 6 in, 2 out]
